vi "AES-InvCipher-BLOCK.vi"(8 "error in (no error)":errorcluster, 10 "Cipher Key":u8[](array[numeric]) format="%02x", 11 "cipher [U8]":u8[](array[numeric]) format="%02x") -> (0 "error out":errorcluster, 3 "plain [U8]":u8[](array[numeric]) format="%02x")   [LabVIEW 2010, in "Encryption.lvlib"]
doc: "Unencrypt a block of U8s that are encrypted with AES.\n\nCAUTION:\nThis VI is not secure, it does not protect the memory of the encryption, key and unencrypted data.\n\n(c) Ton Plomp, 2011\nTHIS SOFTWARE IS PROVIDED AS IS, AND ANY WARRANTY IS REJECTED"
uses:
  Encryption.lvlib
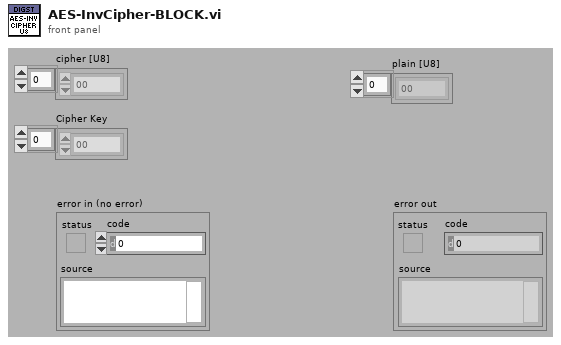
[diagram p1: front panel]
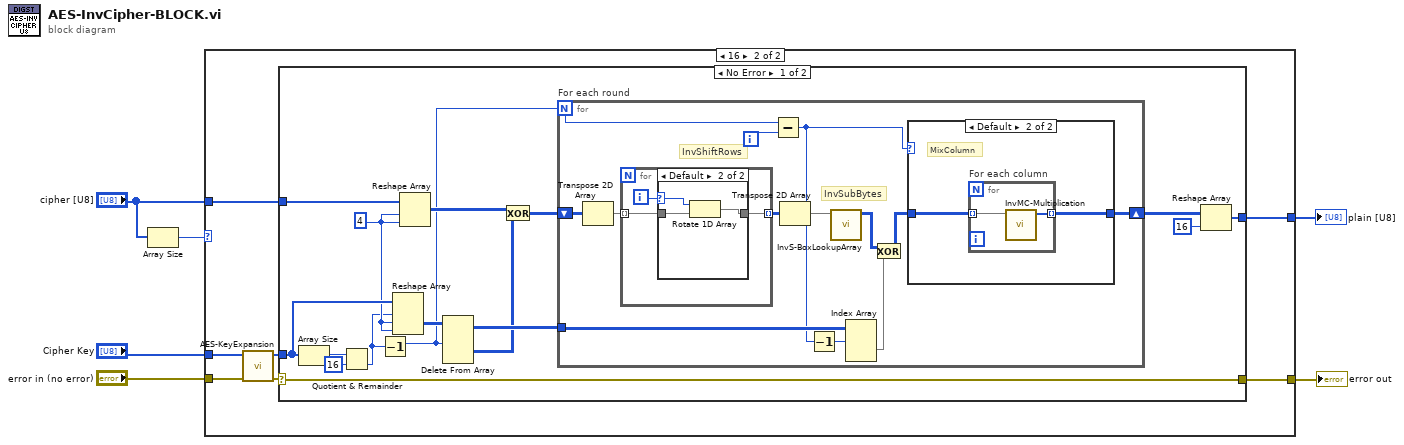
[diagram p0: block diagram]
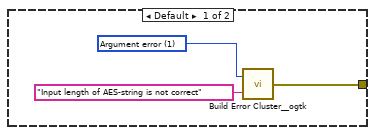
[diagram p2: hidden frame]
diagram:
  n1 = Array Size(array="cipher [U8]") -> (size(s)=w2:i32)
  n2 = case shown="16" w2 {
    tunnel: [_ w15] -> w6
    tunnel: "Cipher Key" -> [_ w14]
    tunnel: "error in (no error)" -> [_ w13]
    tunnel: "cipher [U8]" -> [_ w12]
    tunnel: [w9 w10] -> w1
    frame Default {
      w8 = 1 items=["No error", "Argument error", "Memory is full", "Out of zone", "End of file", "File already open", "Generic file I/O error", "File not found", "File permission error", "Disk is full", "Duplicate path", "Too many files open", "System feature not enabled", "Resource file not found", "Cannot add resource", "Resource not found", "Image not found", "Image memory error", "Pen does not exist", "Config type invalid", "Config token not found", "Config parse error", "Config memory error", "Bad external code format", "Bad external code offset", "External code not present", "Null window", "Destroy window error", "Null menu", "Print aborted", "Bad print record", "Print driver error", "Windows error during printing", "Memory error during printing", "Print dialog error", "Generic print error", "Invalid device refnum", "Device not found", "Device parameter error", "Device unit error", "Cannot open device", "Device call aborted", "Generic error", "Cancelled by user", "Object ID too low", "Object ID too high", "Object not in heap", "Unknown heap", "Unknown object (invalid DefProc)", "Unknown object (DefProc not in table)", "Message out of range", "Invalid (null) method", "Unknown message", "Manager call not supported", "Bad address", "Network operation in progress", "Network operation timed out", "Connection is busy", "Network attribute not supported", "Network error", "Address in use", "System out of memory", "Connection aborted", "Connection refused", "Not connected", "Already connected", "Connection closed", "Initialization error (interapplication manager)", "Bad occurrence", "Wait on unbound occurrence handler", "Occurrence queue overflow", "Datalog type conflict", "Unused", "Unrecognized type (interapplication manager)", "Memory corrupt", "Failed to make temporary DLL", "Old CIN version", "Drag socket not found", "Failed to load drop-object", "Failed to register OLE object", "Failed to release OLE object", "Format specifier type mismatch", "Unknown format specifier", "Too few format specifiers", "Too many format specifiers", "Scan failed", "Newer CIN version", "Error converting to variant", "Runtime menu error", "Password tampered", "Variant attribute not found", "Incompatible variant data type", "Event data is not available", "Event Store is not present", "Occurrence is not found", "Event Queue is not created", "Event info is not available", "Refnum passed is NULL", "Error retrieving Class GUID", "Error retrieving CoClass GUID", "Error retrieving TypeLib GUID.", "Bad built application magic bytes.", "Specific driver is different from the specific driver associated with the Logical Name.", "There is no session opened to the class driver.", "Max Error", "MAX - Error with config objects", "MAX - Error loading configuration", "MAX - Group not supported"]
      n3 = call <userlib>:"Build Error Cluster__ogtk.vi"("String to Prepend to source (\"\")"="Input length of AES-string is not correct" ("String to Prepend to source (\"\")"), "code"=w8) -> ("error out"=w9:errorcluster)
    }
    frame 16 {
      n4 = call "AES-KeyExpansion.vi"("error in (no error)"=w13, "Key In"=w14) -> ("error out"=w11:errorcluster, "Expanded Key [U8]"=w16:u8[])  [unwired: 8 in]
      n5 = case shown="No Error" w11 {
        selector: w11 -> [w21 w58]
        tunnel: w16 -> [w30 _]
        tunnel: [w25 _] -> w15
        tunnel: w12 -> [w23 _]
        tunnel: [w21 w58] -> w10
        frame No Error {
          w22 = 4 ("y")
          n6 = Array Size(array=w30) -> (size(s)=w32:i32)
          n7 = Quotient & Remainder(x=w32, y=16) -> (floor(x/y)=w18:i32)  [unwired: 1 out]
          n8 = Decrement(x=w18) -> (x-1=w17:i32)
          n9 = Reshape Array(w30, w18, w22, w22) -> (w29:u8[][][])
          n10 = Reshape Array(w23, w22, w22) -> (w20:u8[][])
          n11 = Delete From Array(array=w29, index (dim 0)=w17) -> (deleted portion=w19:u8[][], array with subset deleted=w28:u8[][][])  [unwired: 3 in]
          n12 = Exclusive Or(1:w19, 2:w20) -> (0:w27:u8[][])
          n13 = for "For each round" {
            N: w17 -> [w45]
            shift-right: [w33] -> w26
            shift-left: w27 -> [w43]
            tunnel: w28 -> [w38]
            i -> [w44]
            # "InvShiftRows"
            # "InvSubBytes"
            n14 = Transpose 2D Array(2D array=w43) -> (transposed array=w41:u8[][])
            n15 = for {
              tunnel: w41 -> [w52] mode=indexing
              tunnel: [w51] -> w42 mode=indexing
              i -> [w53]
              n16 = case shown="Default" w53 {
                selector: w53 -> [_ w55]
                tunnel: w52 -> [w54 w57]
                tunnel: [w54 w56] -> w51
                frame 0 {
                }
                frame Default {
                  n17 = Rotate 1D Array(1:w57, 2:w55) -> (0:w56:u8[])
                }
              }
            }
            n18 = Subtract(x=w45, y=w44) -> (x-y=w37:i32)
            n19 = Transpose 2D Array(2D array=w42) -> (transposed array=w40:u8[][])
            n20 = Decrement(x=w37) -> (x-1=w36:i32)
            n21 = call "InvS-BoxLookupArray.vi"("In"=w40) -> ("Out"=w39:u8[][])  [unwired: 10 in]
            n22 = Index Array(array=w38, index (dim 0)=w36) -> (element=w35:u8[][])  [unwired: 2 in]
            n23 = Exclusive Or(1:w35, 2:w39) -> (0:w34:u8[][])
            n24 = case shown="Default" w37 {
              tunnel: w34 -> [w46 w48]
              tunnel: [w46 w47] -> w33
              frame 1 {
                # "Last Round"
              }
              frame Default {
                # "MixColumn"
                n25 = for "For each column" {
                  tunnel: w48 -> [w49] mode=indexing
                  tunnel: [w50] -> w47 mode=indexing
                  n26 = call "InvMC-Multiplication.vi"("Vector In"=w49) -> ("Vector Out"=w50:u8[])  [unwired: 10 in]
                }
              }
            }
          }
          n27 = Reshape Array(w26, 16 ("dimension size")) -> (w25:u8[])
        }
        frame Error {
        }
      }
    }
  }
  "error out" <- w1
  "plain [U8]" <- w6
